vi "Network Sink - Log Aggregator.vi"() -> ()   [LabVIEW 2019, in "Network Logger Examples.lvlib"]
uses:
  <vilib>/gpm_packages/@cs/event-logger/Examples/Examples/Network Logger Examples.lvlib
  <vilib>/gpm_packages/@cs/event-logger/Source/Composed Log/LoggerReference/LoggerReference.lvclass/LoggerReference.ctl
  <vilib>/gpm_packages/@cs/event-logger/Source/Composed Log/Types/Log Level.ctl
  b558ab63-4aa2-4cbd-b208-fa7bab295c73.vi
  <vilib>/gpm_packages/@cs/event-logger/Source/Composed Log/LoggerReference/Return Aggregate Queues.vi
  <vilib>/gpm_packages/@cs/event-logger/Source/Composed Log/LoggerReference/Add Aggregate Log.vi
  b558ab63-4aa2-4cbd-b208-fa7bab295c73.vi/7ab4eca4-2d70-4760-ba2d-d04abd9b1f25.vi
  <vilib>/gpm_packages/@cs/event-logger/Source/Composed Log/LoggerReference/Log.vi
  <vilib>/gpm_packages/@cs/event-logger/Source/Composed Log/LoggerReference/Get Valid Event Time.vi
  <vilib>/gpm_packages/@cs/event-logger/Source/Composed Log/LoggerReference/Send Add Sink.vi
  <vilib>/gpm_packages/@cs/event-logger/Source/Composed Log/LoggerReference/Remove Stale Logs.vi
  <vilib>/gpm_packages/@cs/event-logger/Source/String Control Sink/String Control Sink.lvclass
  C:/Program Files/National Instruments/LabVIEW 2019/vi.lib/gpm_packages/@cs/event-logger/Source/Composed Log/Log Sink/Log Sink.lvclass
  <vilib>/gpm_packages/@cs/event-logger/Source/Composed Log/Application Logger/Launch Worker Loop.vi
  <vilib>/gpm_packages/@cs/event-logger/Source/Composed Log/LoggerReference/Initialize Logger Instance.vi
  <vilib>/gpm_packages/@cs/event-logger/Source/Composed Log/LoggerReference/LoggerReference.lvclass
  <vilib>/gpm_packages/@cs/event-logger/Source/Composed Log/IErrorFormat/IErrorFormat.lvclass
  <vilib>/gpm_packages/@cs/event-logger/Source/Composed Log/Log Sink/Log Sink.lvclass
  <vilib>/gpm_packages/@cs/event-logger/Source/Composed Log/Composed Log.lvlib
  <vilib>/gpm_packages/@cs/event-logger/Source/Network Sink/Network Sink Endpoint/Network Sink Endpoint.lvclass
panel:
  in  "Event Level":T1(ring)
  in  "Data To Log":string
  in  "Source":string="User"
  in  "Log":bool
  in  "System Event Log":string
  # "Run the VI. If it isn't already running, start the VIs - Network Sink - Module 1 and Module 2. Use the log custom event to add user defined log messages. Observe that the log aggregator catches events from this module, and the the two remote modules."
  # "Log Custom Event"
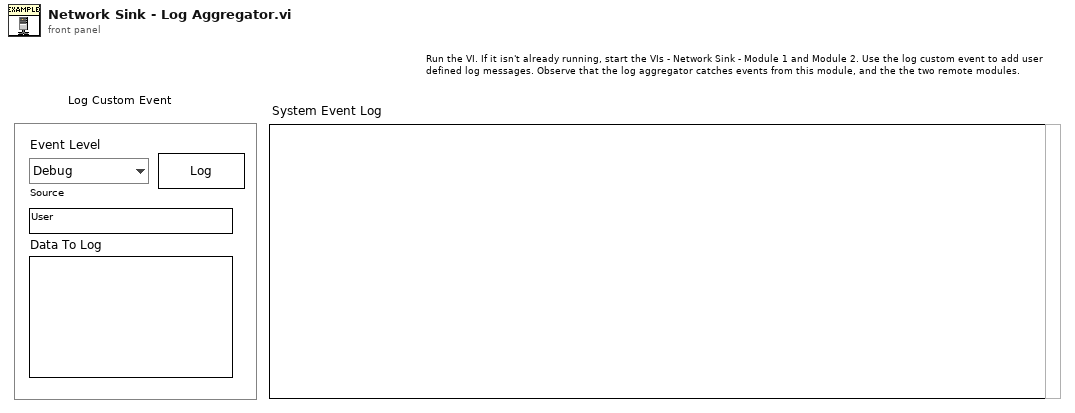
[diagram p1: front panel]
types:
  T1 = enum16{"Debug", "Info", "Warning", "Error", "Critical"}
  T2 = typedef "Composed Log.lvlib/Log Level.ctl" = enum16{"Debug", "Info", "Warning", "Error", "Critical"}
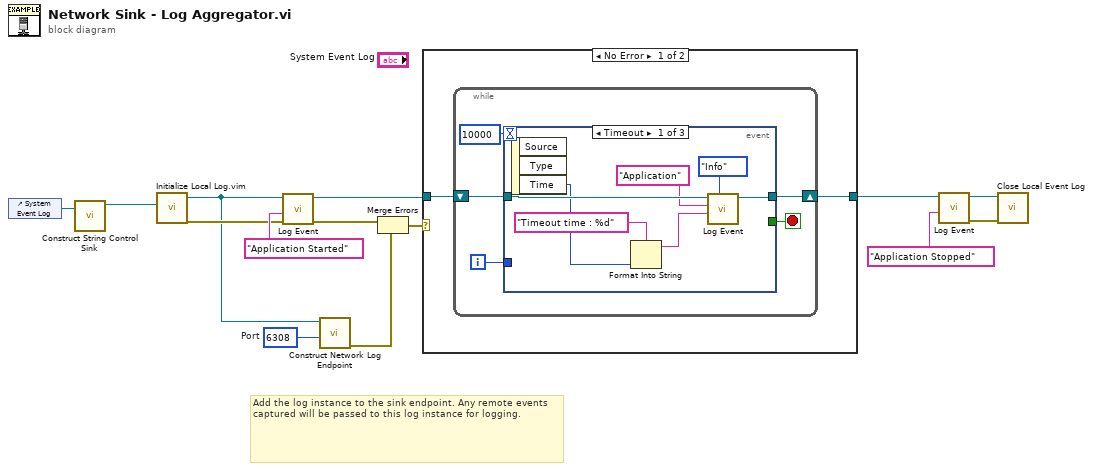
[diagram p0: block diagram]
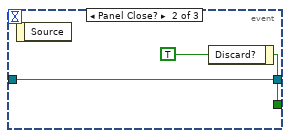
[diagram p2: hidden frame]
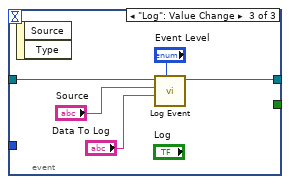
[diagram p3: hidden frame]
diagram:
  w5 = u16 6308  # Port
  # "Add the log instance to the sink endpoint. Any remote events captured will be passed to this log instance for logging."
  n1 = control-ref of="System Event Log"() -> (w14:refnum<vi>)
  n2 = call <vilib>:"Construct String Control Sink.vi"("Str Refnum"=w14) -> ("String Control Sink out"=w1:refnum<class "String Control Sink.lvclass">)  [unwired: 10 in]
  n3 = call "Initialize Local Log.vim"("Startup Sink(s)"=w1) -> ("error out"=w7:errorcluster, "Log Instance Reference"=w4:refnum<class "LoggerReference.lvclass">)  [unwired: 8 in, 1 out]
  n4 = call <vilib>:"Log Event.vi"("error in (no error)"=w7, "Data To Log"="Application Started", "Log Instance"=w4) -> ("error out"=w8:errorcluster, "Log Instance Out"=w9:refnum<class "LoggerReference.lvclass">)  [unwired: 7 in]
  n5 = call <vilib>:"Construct Network Log Endpoint.vi"("Port"=w5, "Logger to Write To"=w4) -> ("error out"=w2:errorcluster)  [unwired: 8 in, 1 out]
  n6 = Merge Errors(w8, w2) -> (w3:errorcluster)
  n7 = case shown="No Error" w3 {
    tunnel: w9 -> [w16 w36]
    tunnel: [w15 w36] -> w13
    frame No Error {
      n8 = while {
        shift-right: [w19] -> w15
        shift-left: w16 -> [w20]
        i -> [w17]
        stop <- w21 stop-if-true
        n9 = event shown="[0] Timeout" {
          selector: _ -> [_ _ _]
          dyn-events: _ -> [_ _ _]
          timeout: 10000 -> [_ _ _]
          tunnel: [_ w30 _] -> w21
          tunnel: w20 -> [w28 w29 w35]
          tunnel: [w26 w29 w33] -> w19
          tunnel: w17 -> [_ _ _]
          event Timeout {
            n10 = event-data() -> ("Time"=w22:u32)  [unwired: 1 in, 2 out]
            n11 = Format Into String(format string="Timeout time : %d" ("Data To Log"), w22) -> (resulting string=w23:string)  [unwired: 2 in, 1 out]
            n12 = call <vilib>:"Log Event.vi"("Event Level"=Log_Level."Info", "Data To Log"=w23, "SourceID"="Application", "Log Instance"=w28) -> ("Log Instance Out"=w26:refnum<class "LoggerReference.lvclass">)  [unwired: 6 in, 1 out]
          }
          event Panel Close? {
            w30 = TRUE ("Discard?")
            n13 = event-data() -> ()  [unwired: 1 in, 1 out]
            n14 = event-data("Discard?"=w30) -> ()  [unwired: 1 in, 1 out]
          }
          event "Log": Value Change {
            n15 = event-data() -> ()  [unwired: 1 in, 2 out]
            n16 = call <vilib>:"Log Event.vi"("Event Level"="Event Level", "Data To Log"="Data To Log", "SourceID"="Source", "Log Instance"=w35) -> ("Log Instance Out"=w33:refnum<class "LoggerReference.lvclass">)  [unwired: 6 in, 1 out]
          }
        }
      }
    }
    frame Error {
    }
  }
  n17 = call <vilib>:"Log Event.vi"("Data To Log"="Application Stopped", "Log Instance"=w13) -> ("error out"=w6:errorcluster, "Log Instance Out"=w12:refnum<class "LoggerReference.lvclass">)  [unwired: 8 in]
  n18 = call <vilib>:"Close Local Event Log.vi"("error in (no error)"=w6, "Log Instance"=w12) -> ()  [unwired: 9 in, 1 out]
